vi "_TBD Get Date-Time String.vi"() -> (0 "Current Time Stamp (now timestamp)":timestamp, 1 "Date-Time String":string)   [LabVIEW 2023, in "Error Manager.lvlib" / "Error Log.lvclass"]
uses:
  Error Log.lvclass
  Error Log.lvclass/Error Log.ctl
panel:
  # "Input\nInputs to the VI"
  # "Development\nControls or indicators that are useful for development or testing, but which are not outputs of the VI."
  # "Output\nOutputs of the VI"
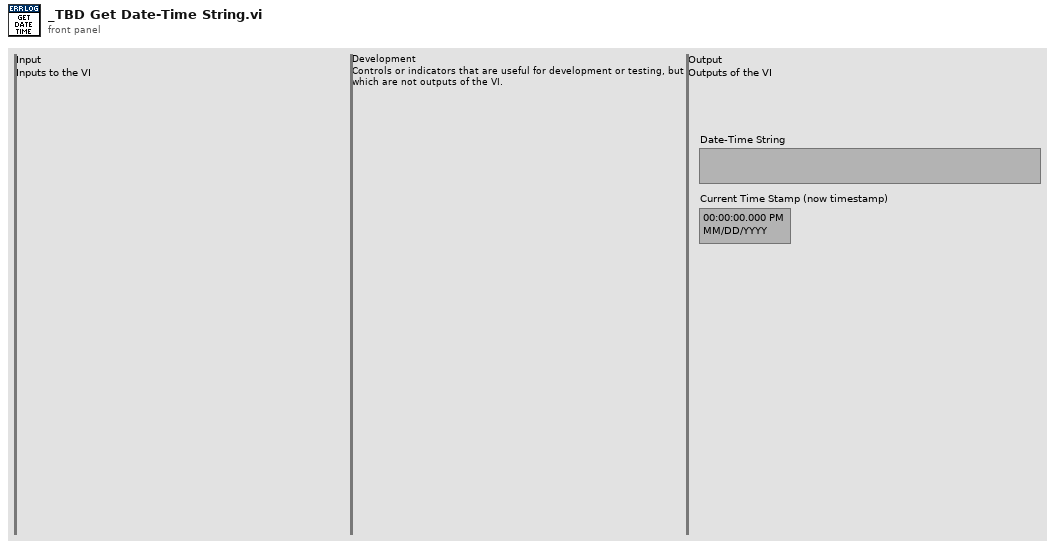
[diagram p1: front panel]
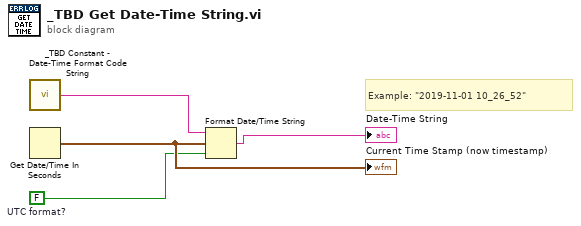
[diagram p0: block diagram]
diagram:
  w1 = FALSE  # UTC format?
  # "Example: \"2019-11-01 10_26_52\""
  n1 = call "_TBD Constant - Date-Time Format Code String.vi"() -> ("Date-Time Format String"=w3:string)
  n2 = Get Date/Time In Seconds() -> (seconds since 1Jan1904=w2:timestamp)
  "Current Time Stamp (now timestamp)" <- w2
  n3 = Format Date/Time String(time format string (%c)=w3, seconds (now)=w2, UTC format=w1) -> (date/time string=→"Date-Time String":string)
